vi "move to take ball 1.vi"   [LabVIEW 2016, in "Test2.lvrbt"]
uses:
  Test2.lvrbt
  <vilib>/NXT/Block Support/NXT_InputPort.ctl
  <vilib>/NXT/Hardware/Plugins/Tetrix DC Motor/TetrixDCMotorAddress.ctl
  <vilib>/NXT/NXTIO Xnodes/NXTIONodeSubVIs/TETRIX IO Move DC Motors.vi
  <vilib>/NXT/Dual Mode Library/Waits/Wait_EV3_Ultrasonic_Centimeters_Further.vi
  <vilib>/NXT/NXTIO Xnodes/NXTIONodeSubVIs/TETRIX IO Stop DC Motors.vi
  <vilib>/NXT/Dual Mode Library/Waits/Wait_Num.vi
  <vilib>/NXT/Dual Mode Library/Waits/Wait_EV3_Ultrasonic_Centimeter_Closer.vi
  <vilib>/NXT/Subs/LVHSConnector.ctl
  <vilib>/NXT/NXTIO Xnodes/AddressXNode/NXTIOAddress.xnode
  <vilib>/NXT/NXTIO Xnodes/NXTIOXNode/NXTIO.xnode
  <vilib>/NXT/LegoClasses/BrickReference/BrickReference.lvclass
types:
  T1 = typedef "NXT_InputPort.ctl" = u32
  T2 = typedef "TetrixDCMotorAddress.ctl" = i32
  T3 = typedef "LVHSConnector.ctl" = refnum<class "BrickReference.lvclass">
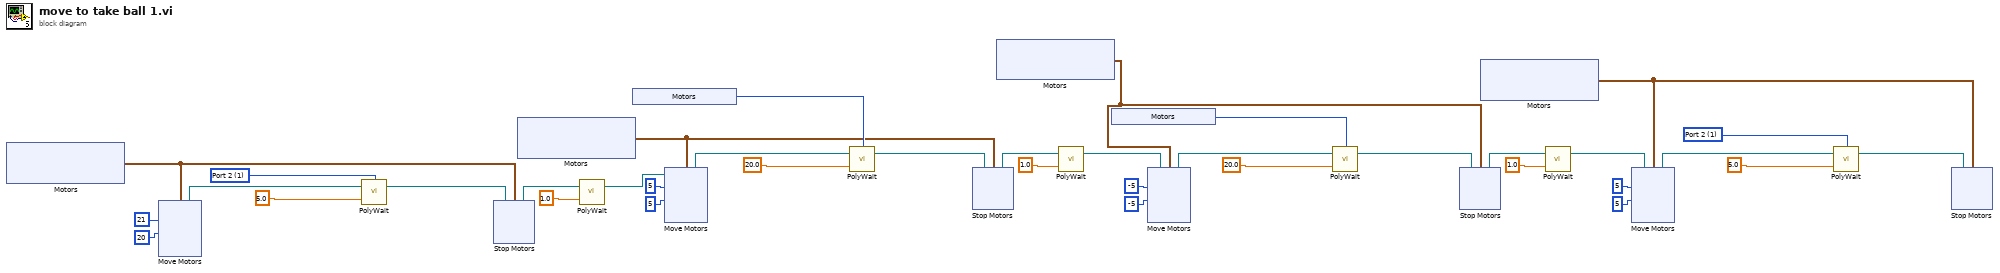
[diagram p0: block diagram]
diagram:
  w3 = T1 1 items=["Port 1", "Port 2", "Port 3", "Port 4"] ("Port (Port 1)")
  w29 = T1 1 items=["Port 1", "Port 2", "Port 3", "Port 4"] ("Port (Port 1)")
  n1 = xnode "Motors"() -> ("Motor"=w32:cluster{"TetrixDCMotor":T2, "TetrixDCMotor":T2})
  n2 = xnode "Move Motors"("Power/Speed 2"=i8 20, "Power/Speed 1"=i8 21, "Motors"=w32) -> ("NXT/EV3"=w35:T3)  [unwired: 1 in]
  n3 = call-poly <vilib>:"PolyWait.vi"("Centimeters (50)"=sgl 5.0, "NXT/EV3"=w35, "Port (Port 1)"=w29) -> ("NXT/EV3"=w33:T3)  [unwired: 1 in]
  n4 = xnode "Stop Motors"("Motors"=w32, "NXT/EV3"=w33) -> ("NXT/EV3"=w30:T3)
  n5 = xnode "Motors"() -> ("Motor"=w22:cluster{"TetrixDCMotor":T2, "TetrixDCMotor":T2})
  n6 = call-poly <vilib>:"PolyWait.vi"("Time (1 sec)"=sgl 1.0, "NXT/EV3"=w30) -> ("NXT/EV3"=w21:T3)  [unwired: 2 in]
  n7 = xnode "Motors"() -> ("Sensor"=w24:T1)
  n8 = xnode "Move Motors"("Power/Speed 2"=i8 5, "Power/Speed 1"=i8 5, "Motors"=w22, "NXT/EV3"=w21) -> ("NXT/EV3"=w26:T3)
  n9 = call-poly <vilib>:"PolyWait.vi"("Centimeters (40)"=sgl 20.0, "NXT/EV3"=w26, "Port (Port 1)"=w24) -> ("NXT/EV3"=w23:T3)  [unwired: 1 in]
  n10 = xnode "Stop Motors"("Motors"=w22, "NXT/EV3"=w23) -> ("NXT/EV3"=w20:T3)
  n11 = xnode "Motors"() -> ("Motor"=w13:cluster{"TetrixDCMotor":T2, "TetrixDCMotor":T2})
  n12 = call-poly <vilib>:"PolyWait.vi"("Time (1 sec)"=sgl 1.0, "NXT/EV3"=w20) -> ("NXT/EV3"=w16:T3)  [unwired: 2 in]
  n13 = xnode "Motors"() -> ("Sensor"=w11:T1)
  n14 = xnode "Move Motors"("Power/Speed 2"=i8 -5, "Power/Speed 1"=i8 -5, "Motors"=w13, "NXT/EV3"=w16) -> ("NXT/EV3"=w15:T3)
  n15 = call-poly <vilib>:"PolyWait.vi"("Centimeters (50)"=sgl 20.0, "NXT/EV3"=w15, "Port (Port 1)"=w11) -> ("NXT/EV3"=w14:T3)  [unwired: 1 in]
  n16 = xnode "Stop Motors"("Motors"=w13, "NXT/EV3"=w14) -> ("NXT/EV3"=w9:T3)
  n17 = xnode "Motors"() -> ("Motor"=w1:cluster{"TetrixDCMotor":T2, "TetrixDCMotor":T2})
  n18 = call-poly <vilib>:"PolyWait.vi"("Time (1 sec)"=sgl 1.0, "NXT/EV3"=w9) -> ("NXT/EV3"=w6:T3)  [unwired: 2 in]
  n19 = xnode "Move Motors"("Power/Speed 2"=i8 5, "Power/Speed 1"=i8 5, "Motors"=w1, "NXT/EV3"=w6) -> ("NXT/EV3"=w5:T3)
  n20 = call-poly <vilib>:"PolyWait.vi"("Centimeters (50)"=sgl 5.0, "NXT/EV3"=w5, "Port (Port 1)"=w3) -> ("NXT/EV3"=w2:T3)  [unwired: 1 in]
  n21 = xnode "Stop Motors"("Motors"=w1, "NXT/EV3"=w2) -> ()  [unwired: 1 out]
